vi "Get Segmented Log Type.vi"(8 "error in (no error)":errorcluster, 11 "Segmented Log in":refnum<class "Segmented Log.lvclass">) -> (0 "error out":errorcluster, 2 "Segmented Log Type":T1, 3 "Segmented Log out":refnum<class "Segmented Log.lvclass">)   [LabVIEW 2015, in "Segmented Log.lvclass"]
uses:
  Segmented Log.lvclass
  Segmented Log Type.ctl
  Segmented Log.lvclass/Segmented Log.ctl
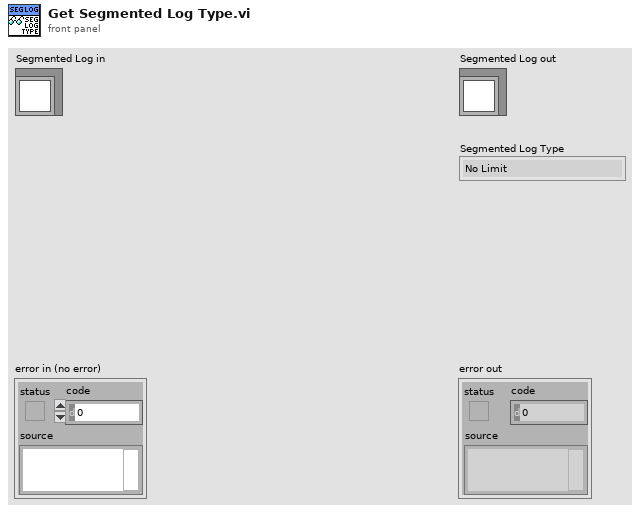
[diagram p1: front panel]
types:
  T1 = typedef "Segmented Log.lvclass/Segmented Log Type.ctl" = enum16{"No Limit", "Footprint", "Time"}
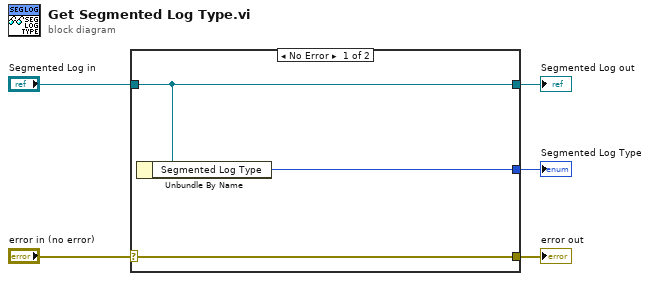
[diagram p0: block diagram]
diagram:
  n1 = case shown="No Error" "error in (no error)" {
    selector: "error in (no error)" -> [w8 w9]
    tunnel: [w8 w9] -> w4
    tunnel: [w7 w10] -> w2
    tunnel: "Segmented Log in" -> [w7 w10]
    tunnel: [w6 _] -> w1
    frame No Error {
      n2 = Unbundle By Name(w7) -> ("Segmented Log Type"=w6:T1)
    }
    frame Error {
    }
  }
  "error out" <- w4
  "Segmented Log out" <- w2
  "Segmented Log Type" <- w1
